vi "Vision - Get Sections.vi"(4 "Page":u8, 6 "Vision Settings":T1 {"Dist/Page" items=["Blue (M)/Black (C)", "Red (M)/Green (C)"]}, 7 "Current Pos (km)":dbl, 8 "error in (no error)":errorcluster, 10 "Inc/page (km)":dbl) -> (0 "error out":errorcluster, 2 "Sections Out":T3[](array[typedef]))   [LabVIEW 2024]
uses:
  Controls/Vision - Section.ctl
  Buttons/Bin.ctl
  Controls/Vision - Reporting Settings.ctl
  Controls/Vision - Dist Per Page.ctl
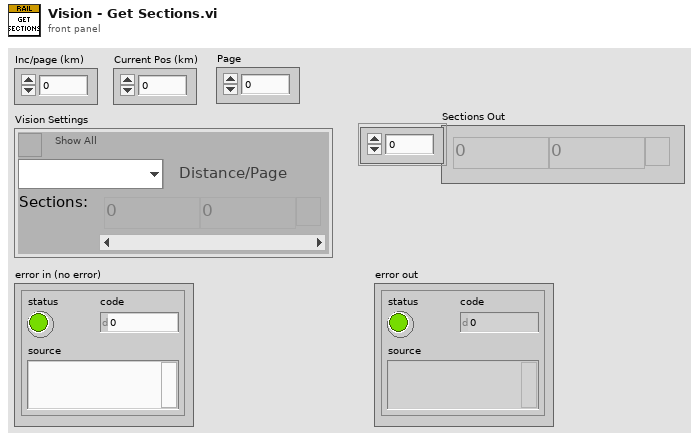
[diagram p1: front panel]
types:
  T1 = typedef "Vision - Reporting Settings.ctl" = cluster{"Show All?":bool, "Dist/Page":T2, "Sections":T3[]}
  T2 = typedef "Vision - Dist Per Page.ctl" = u16
  T3 = typedef "Vision - Section.ctl" = cluster{"From":dbl, "To":dbl, "Discard":T4}
  T4 = typedef "Bin.ctl" = bool
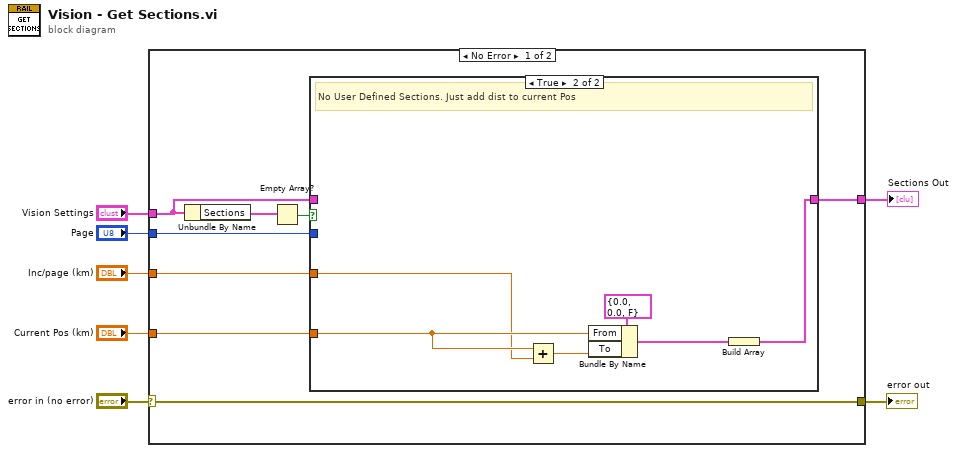
[diagram p0: block diagram]
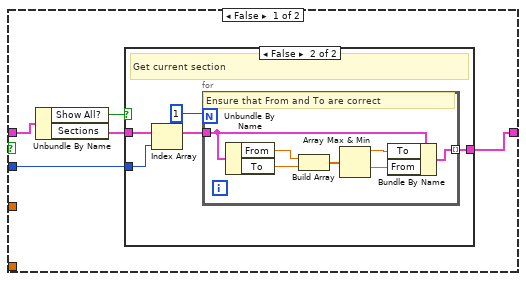
[diagram p2: hidden frame]
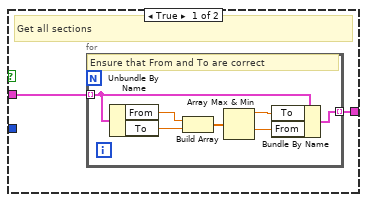
[diagram p3: hidden frame]
diagram:
  n1 = case shown="No Error" "error in (no error)" {
    selector: "error in (no error)" -> [w15 w48]
    tunnel: [w15 w48] -> w6
    tunnel: "Inc/page (km)" -> [w12 _]
    tunnel: "Vision Settings" -> [w9 _]
    tunnel: "Current Pos (km)" -> [w13 _]
    tunnel: [w11 _] -> w3
    tunnel: "Page" -> [w8 _]
    frame No Error {
      n2 = Unbundle By Name(w9) -> ("Sections"=w10:T3[])
      n3 = Empty Array?(array=w10) -> (empty?=w14:bool)
      n4 = case shown="True" w14 {
        tunnel: w13 -> [_ w45]
        tunnel: w12 -> [_ w44]
        tunnel: w9 -> [w20 _]
        tunnel: [w19 w42] -> w11
        tunnel: w8 -> [w16 _]
        frame False {
          n5 = Unbundle By Name(w20) -> ("Show All?"=w17:bool, "Sections"=w18:T3[])
          n6 = case shown="False" w17 {
            tunnel: [w22 w34] -> w19
            tunnel: w18 -> [w21 w33]
            tunnel: w16 -> [_ w31]
            frame True {
              # "Get all sections"
              n7 = for {
                tunnel: w21 -> [w26] mode=indexing
                tunnel: [w23] -> w22 mode=indexing
                # "Ensure that From and To are correct"
                n8 = Unbundle By Name(w26) -> ("From"=w29:dbl, "To"=w28:dbl)
                n9 = Build Array(w29, w28) -> (w27:dbl[])
                n10 = Array Max & Min(array=w27) -> (max value=w25:dbl, min value=w24:dbl)  [unwired: 2 out]
                n11 = Bundle By Name(cluster=w26, "To"=w25, "From"=w24) -> (w23:T3)
              }
            }
            frame False {
              # "Get current section"
              n12 = Index Array(array=w33, index=w31) -> (element=w32:T3)
              n13 = for {
                N: 1 -> [_]
                tunnel: w32 -> [w38]
                tunnel: [w35] -> w34 mode=indexing
                # "Ensure that From and To are correct"
                n14 = Unbundle By Name(w38) -> ("From"=w41:dbl, "To"=w40:dbl)
                n15 = Build Array(w41, w40) -> (w39:dbl[])
                n16 = Array Max & Min(array=w39) -> (max value=w37:dbl, min value=w36:dbl)  [unwired: 2 out]
                n17 = Bundle By Name(cluster=w38, "To"=w37, "From"=w36) -> (w35:T3)
              }
            }
          }
        }
        frame True {
          # "No User Defined Sections. Just add dist to current Pos"
          n18 = Add(x=w45, y=w44) -> (x+y=w46:dbl)
          n19 = Bundle By Name(cluster=T3 {"From"=0.0, "To"=0.0, "Discard"=FALSE} ("Sections"), "From"=w45, "To"=w46) -> (w43:T3)
          n20 = Build Array(w43) -> (w42:T3[])
        }
      }
    }
    frame Error {
    }
  }
  "error out" <- w6
  "Sections Out" <- w3
